vi "Parse Signal List.vi"(8 "error in":errorcluster, 11 "PRM in":refnum<class "PRM.lvclass">) -> (0 "error out":errorcluster, 3 "PRM out":refnum<class "PRM.lvclass">)   [LabVIEW 2019, in "PRM.lvlib" / "PRM.lvclass"]
uses:
  Library/PRM.lvclass
  C:/Users/Public/Documents/Development/builds/Tools/Config.lvlibp/Config.lvclass
  Custom Controls/Signal List Keys.ctl
  Library/PRM.lvclass/PRM.ctl
  builds/Tools/Config.lvlibp/Accessors/Read Device Signals.vi
panel:
  in  "Signal List Keys":T1=enum."NAME"
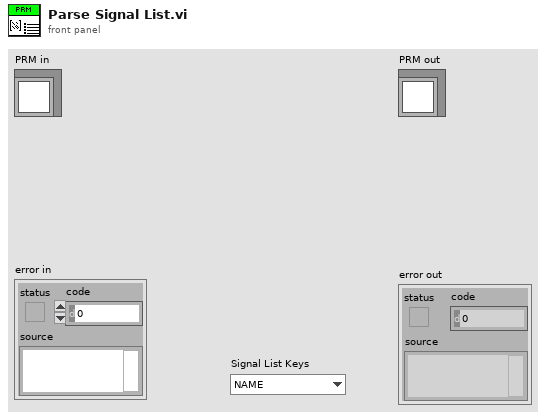
[diagram p1: front panel]
types:
  T1 = typedef "PRM.lvlib/PRM.lvclass/Signal List Keys.ctl" = enum16{"PIN", "NAME", "MAX", "MIN", "RTD_A", "RTD_B", "RTD_C", "RTD_R0"}
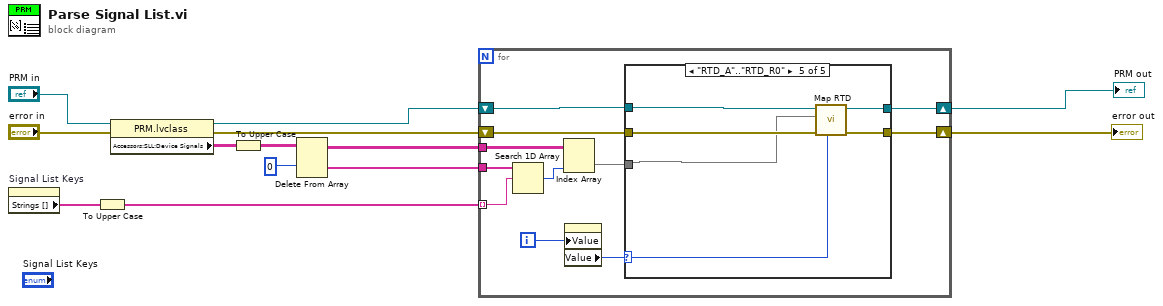
[diagram p0: block diagram]
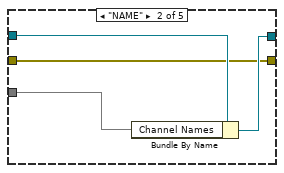
[diagram p3: hidden frame]
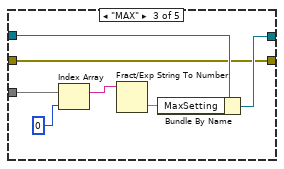
[diagram p4: hidden frame]
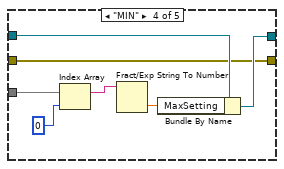
[diagram p5: hidden frame]
diagram:
  n1 = property on="Signal List Keys" class="Enum (strict)"() -> ("Strings []"=w8:string[])  [unwired: 2 in, 2 out]
  n2 = To Upper Case(1:w8) -> (0:w3:string[])
  n3 = property class="PRM.lvclass"(reference="PRM in", error in="error in") -> (reference out=w7:refnum<class "PRM.lvclass">, error out=w5:errorcluster, "Accessors:SLL:Device Signals"=w12:string[][])
  n4 = To Upper Case(1:w12) -> (0:w9:string[][])
  n5 = Delete From Array(array=w9, index (row)=0 ("disabled index (col)")) -> (deleted portion=w2:string[], array with subset deleted=w1:string[][])  [unwired: 2 in]
  n6 = for {
    tunnel: w3 -> [w17] mode=indexing
    shift-right: [w21] -> w6
    shift-left: w7 -> [w22]
    shift-right: [w19] -> w4
    shift-left: w5 -> [w20]
    tunnel: w2 -> [w18]
    tunnel: w1 -> [w14]
    i -> [w24]
    n7 = Search 1D Array(1D array=w18, element=w17) -> (index of element=w16:i32)  [unwired: 1 in]
    n8 = Index Array(array=w14, index (col)=w16) -> (element=w15:string[])  [unwired: 1 in]
    n9 = property on="Signal List Keys" class="Enum (strict)"("Value"=w24) -> ("Value"=w23:T1)  [unwired: 2 in, 2 out]
    n10 = case shown="\"RTD_A\"..\"RTD_R0\"" w23 {
      selector: w23 -> [_ _ _ _ w48]
      tunnel: w22 -> [w26 w30 w37 w44 w50]
      tunnel: [w26 w29 w36 w42 w49] -> w21
      tunnel: w20 -> [w25 w28 w35 w41 w47]
      tunnel: [w25 w28 w35 w41 w46] -> w19
      tunnel: w15 -> [_ w27 w34 w40 w45]
      frame "PIN" {
      }
      frame "NAME" {
        n11 = Bundle By Name(cluster=w30, "Channel Names"=w27) -> (w29:refnum<class "PRM.lvclass">)
      }
      frame "MAX" {
        n12 = Index Array(array=w34, index=0 ("disabled index (row)")) -> (element=w32:string)
        n13 = Fract/Exp String To Number(string=w32) -> (number=w33:dbl)  [unwired: 3 in, 1 out]
        n14 = Bundle By Name(cluster=w37, "MaxSetting"=w33) -> (w36:refnum<class "PRM.lvclass">)
      }
      frame "MIN" {
        n15 = Index Array(array=w40, index=0 ("disabled index (row)")) -> (element=w39:string)
        n16 = Fract/Exp String To Number(string=w39) -> (number=w43:dbl)  [unwired: 3 in, 1 out]
        n17 = Bundle By Name(cluster=w44, "MaxSetting"=w43) -> (w42:refnum<class "PRM.lvclass">)
      }
      frame "RTD_A".."RTD_R0" {
        n18 = call "Map RTD.vi"("Signal List Keys"=w48, "error in"=w47, "RTD_String"=w45, "PRM in"=w50) -> ("error out"=w46:errorcluster, "PRM out"=w49:refnum<class "PRM.lvclass">)  [unwired: 6 in]
      }
    }
  }
  "PRM out" <- w6
  "error out" <- w4
